vi "Variant To Data - Generic - Scalar.vi"(8 "Error In":errorcluster, 10 "Type code":i32, 11 "Variant":variant) -> (0 "Error Out":errorcluster, 3 "Scalar variable":dbl)   [LabVIEW 2014]
doc: "<B>Copyright</B>: (c) MHWirth 2015. All rights are reserved.\n\nThis SubVI converts variant data (scalars) to doubles. \n\nSupported shared variable types:\nCode 1. Boolean\nCode 2 to 5. Int8/16/32/64\nCode 6 to 9. UInt8/16/32/64\nCode 10. Double\nCode 11. Single-precision\nCode 12. String\nCode 13-23 - 1D array of above types except string\n\n<B>Error 7001</B>: Unknown Data Type - Type Code Array (Int32) contains -1 indicating an unknown data type."
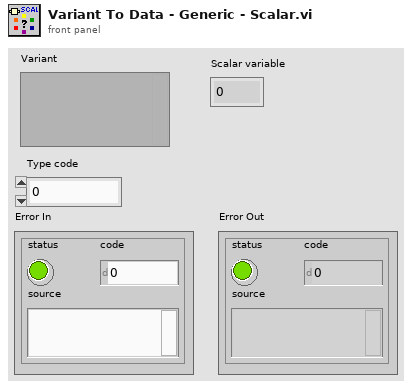
[diagram p1: front panel]
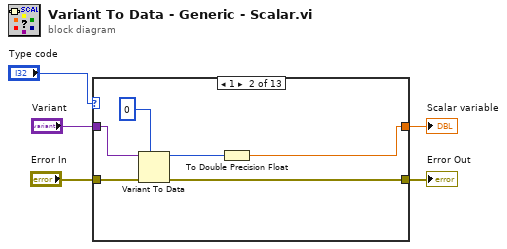
[diagram p0: block diagram]
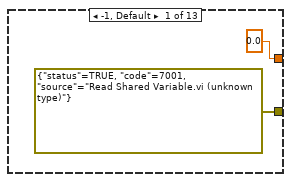
[diagram p2: hidden frame]
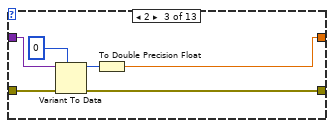
[diagram p3: hidden frame]
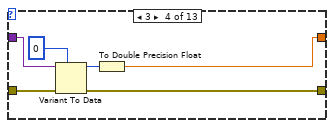
[diagram p4: hidden frame]
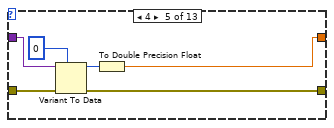
[diagram p5: hidden frame]
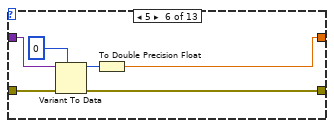
[diagram p6: hidden frame]
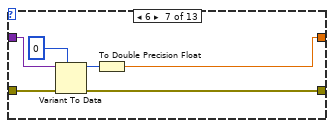
[diagram p7: hidden frame]
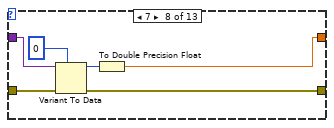
[diagram p8: hidden frame]
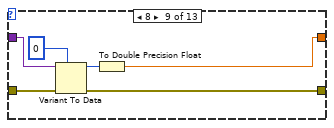
[diagram p9: hidden frame]
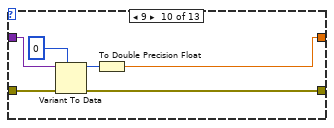
[diagram p10: hidden frame]
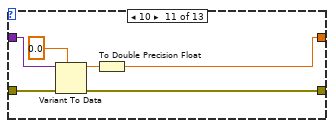
[diagram p11: hidden frame]
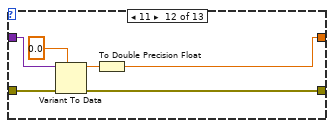
[diagram p12: hidden frame]
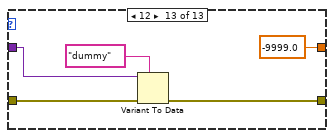
[diagram p13: hidden frame]
diagram:
  n1 = case shown="1" "Type code" {
    tunnel: [errorcluster {"status"=TRUE, "code"=7001, "source"="Read Shared Variable.vi (unknown type)"} ("error constant") w13 w19 w25 w31 w37 w43 w49 w55 w61 w67 w73 w78] -> w5
    tunnel: "Error In" -> [_ w12 w18 w24 w30 w36 w42 w48 w54 w60 w66 w72 w77]
    tunnel: [0.0 w10 w14 w20 w26 w32 w38 w44 w50 w56 w62 w68 -9999.0] -> w1
    tunnel: "Variant" -> [_ w11 w15 w22 w27 w33 w39 w45 w51 w57 w63 w69 w75]
    frame -1, Default {
    }
    frame 1 {
      n2 = Variant To Data(error in=w12, type=i16 0 ("0, 1"), Variant=w11) -> (data=w8:i16, error out=w13:errorcluster)
      n3 = To Double Precision Float(number=w8) -> (double precision float=w10:dbl)
    }
    frame 2 {
      n4 = Variant To Data(error in=w18, type=i8 0, Variant=w15) -> (data=w17:i8, error out=w19:errorcluster)
      n5 = To Double Precision Float(number=w17) -> (double precision float=w14:dbl)
    }
    frame 3 {
      n6 = Variant To Data(error in=w24, type=i16 0, Variant=w22) -> (data=w23:i16, error out=w25:errorcluster)
      n7 = To Double Precision Float(number=w23) -> (double precision float=w20:dbl)
    }
    frame 4 {
      n8 = Variant To Data(error in=w30, type=0, Variant=w27) -> (data=w29:i32, error out=w31:errorcluster)
      n9 = To Double Precision Float(number=w29) -> (double precision float=w26:dbl)
    }
    frame 5 {
      n10 = Variant To Data(error in=w36, type=i64 0, Variant=w33) -> (data=w35:i64, error out=w37:errorcluster)
      n11 = To Double Precision Float(number=w35) -> (double precision float=w32:dbl)
    }
    frame 6 {
      n12 = Variant To Data(error in=w42, type=u8 0, Variant=w39) -> (data=w41:u8, error out=w43:errorcluster)
      n13 = To Double Precision Float(number=w41) -> (double precision float=w38:dbl)
    }
    frame 7 {
      n14 = Variant To Data(error in=w48, type=u16 0, Variant=w45) -> (data=w47:u16, error out=w49:errorcluster)
      n15 = To Double Precision Float(number=w47) -> (double precision float=w44:dbl)
    }
    frame 8 {
      n16 = Variant To Data(error in=w54, type=u32 0, Variant=w51) -> (data=w53:u32, error out=w55:errorcluster)
      n17 = To Double Precision Float(number=w53) -> (double precision float=w50:dbl)
    }
    frame 9 {
      n18 = Variant To Data(error in=w60, type=u64 0, Variant=w57) -> (data=w59:u64, error out=w61:errorcluster)
      n19 = To Double Precision Float(number=w59) -> (double precision float=w56:dbl)
    }
    frame 10 {
      n20 = Variant To Data(error in=w66, type=0.0, Variant=w63) -> (data=w65:dbl, error out=w67:errorcluster)
      n21 = To Double Precision Float(number=w65) -> (double precision float=w62:dbl)
    }
    frame 11 {
      n22 = Variant To Data(error in=w72, type=sgl 0.0, Variant=w69) -> (data=w71:sgl, error out=w73:errorcluster)
      n23 = To Double Precision Float(number=w71) -> (double precision float=w68:dbl)
    }
    frame 12 {
      n24 = Variant To Data(error in=w77, type="dummy", Variant=w75) -> (error out=w78:errorcluster)  [unwired: 1 out]
    }
  }
  "Error Out" <- w5
  "Scalar variable" <- w1
